vi "STEPINDICATOR_091_2.vi"(0 "current step":dbl, 5 "enable":i16, 7 "Reset":bool, 9 "manual":dbl) -> (1 "Led 8":bool, 2 "Led 10":bool, 3 "Led 11":bool, 4 "Led 7":bool, 6 "Led 1":bool, 8 "Led 6":bool, 10 "Led 2":bool, 11 "Led 12":bool, 12 "Led 5":bool, 13 "Led 4":bool, 14 "Led 3":bool, 15 "Led 9":bool)   [LabVIEW 2016]
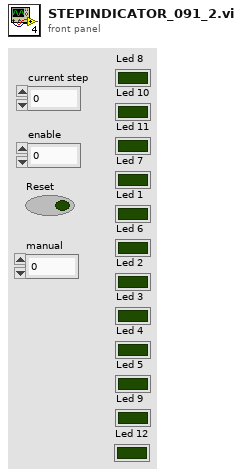
[diagram p1: front panel]
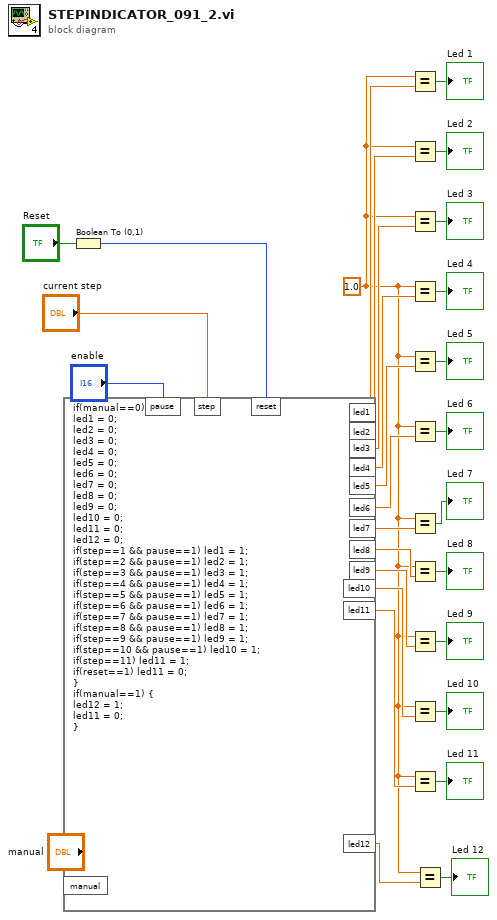
[diagram p0: block diagram]
diagram:
  w1 = 1.0 ("x")
  n1 = Boolean To (0,1)(Boolean="Reset") -> (0, 1=w17:i16)
  n2 = formula code="if(manual==0) {\nled1 = 0;\nled2 = 0;\nled3 = 0;\nled4 = 0;\nled5 = 0;\nled6 = 0;\nled7 = 0;\nled8 = 0;\nled9 = 0;\nled10 = 0;\nled11 = 0;\nled12 = 0;\nif(step==1 && pause==1) led1 = 1;\nif(step==2 && pause==1) led2 = 1;\nif(step==3 && pause==1) led3 = 1;\nif(step==4 && pause==1) led4 = 1;\nif(step==5 && pause==1) led5 = 1;\nif(step==6 && pause==1) led6 = 1;\nif(step==7 && pause==1) led7 = 1;\nif(step==8 && pause==1) led8 = 1;\nif(step==9 && pause==1) led9 = 1;\nif(step==10 && pause==1) led10 = 1;\nif(step==11) led11 = 1;\nif(reset==1) led11 = 0;\n}\nif(manual==1) {\nled12 = 1;\nled11 = 0;\n}"("step"="current step", "pause"="enable", "reset"=w17, "manual"="manual") -> ("led1"=w15:dbl, "led2"=w14:dbl, "led3"=w13:dbl, "led4"=w12:dbl, "led5"=w11:dbl, "led6"=w10:dbl, "led7"=w9:dbl, "led8"=w8:dbl, "led9"=w7:dbl, "led10"=w6:dbl, "led11"=w5:dbl, "led12"=w2:dbl)
  n3 = Equal?(x=w1, y=w15) -> (x = y?=→"Led 1":bool)
  n4 = Equal?(x=w1, y=w14) -> (x = y?=→"Led 2":bool)
  n5 = Equal?(x=w1, y=w13) -> (x = y?=→"Led 3":bool)
  n6 = Equal?(x=w1, y=w12) -> (x = y?=→"Led 4":bool)
  n7 = Equal?(x=w1, y=w11) -> (x = y?=→"Led 5":bool)
  n8 = Equal?(x=w1, y=w10) -> (x = y?=→"Led 6":bool)
  n9 = Equal?(x=w1, y=w9) -> (x = y?=→"Led 7":bool)
  n10 = Equal?(x=w1, y=w8) -> (x = y?=→"Led 8":bool)
  n11 = Equal?(x=w1, y=w7) -> (x = y?=→"Led 9":bool)
  n12 = Equal?(x=w1, y=w6) -> (x = y?=→"Led 10":bool)
  n13 = Equal?(x=w1, y=w5) -> (x = y?=→"Led 11":bool)
  n14 = Equal?(x=w1, y=w2) -> (x = y?=→"Led 12":bool)
